vi "Copy 7zS2SFX.vi"(8 "error in (no error)":errorcluster, 11 "PostBuildSupport in":refnum<class "PostBuildSupport.lvclass">) -> (0 "error out":errorcluster, 3 "PostBuildSupport out":refnum<class "PostBuildSupport.lvclass">)   [LabVIEW 2016, in "PostBuildSupport.lvclass"]
uses:
  PostBuildSupport.lvclass
  PostBuildSupport.lvclass/PostBuildSupport.ctl
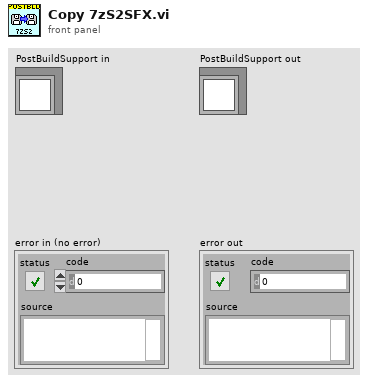
[diagram p1: front panel]
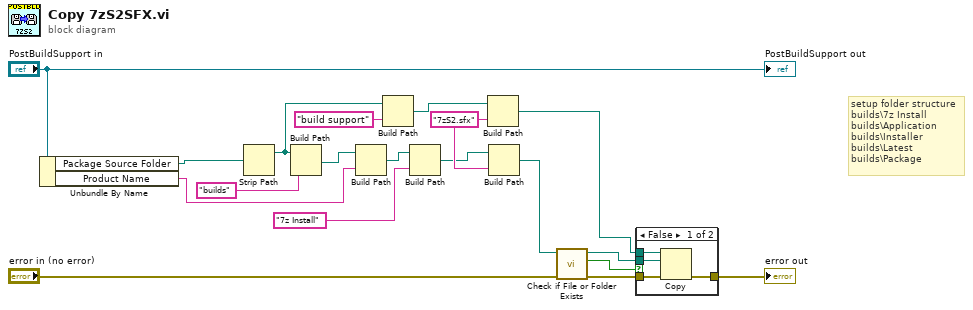
[diagram p0: block diagram]
diagram:
  w9 = "7zS2.sfx" ("name or relative path")
  # "setup folder structure\nbuilds\\7z Install\nbuilds\\Application\nbuilds\\Installer\nbuilds\\Latest\nbuilds\\Package"
  n1 = Unbundle By Name("PostBuildSupport in") -> ("Package Source Folder"=w16:path, "Product Name"=w15:string)
  n2 = Strip Path(path=w16) -> (stripped path=w10:path)  [unwired: 1 out]
  n3 = Build Path(base path=w10, name or relative path="builds") -> (appended path=w18:path)
  n4 = Build Path(base path=w18, name or relative path=w15) -> (appended path=w12:path)
  n5 = Build Path(base path=w10, name or relative path="build support") -> (appended path=w13:path)
  n6 = Build Path(base path=w12, name or relative path="7z Install") -> (appended path=w8:path)
  n7 = Build Path(base path=w13, name or relative path=w9) -> (appended path=w3:path)
  n8 = Build Path(base path=w8, name or relative path=w9) -> (appended path=w4:path)
  n9 = call <vilib>:"Check if File or Folder Exists.vi"("error in (no error)"="error in (no error)", "path"=w4) -> ("error out"=w6:errorcluster, "file or folder exists?"=w5:bool, "dup path"=w7:path)  [unwired: 7 in]
  n10 = case shown="False" w5 {
    tunnel: [w23 w24] -> w2
    tunnel: w3 -> [w22 _]
    tunnel: w7 -> [w21 _]
    tunnel: w6 -> [w20 w24]
    frame False {
      n11 = Copy(8:w20, 10:w21, 11:w22) -> (0:w23:errorcluster)  [unwired: 2 in, 2 out]
    }
    frame True {
    }
  }
  "error out" <- w2
  "PostBuildSupport out" <- "PostBuildSupport in"
